vi "LabVIEW Final Project standard.vi"() -> ()   [LabVIEW 2022 SP3]
uses:
  <vilib>/sound2/lvsound2.llb/Sampling Mode.ctl
  <vilib>/Analysis/2dsp.llb/Real FFT.vi
  <vilib>/sound2/lvsound2.llb/Sound Input Read (DBL).vi
  <vilib>/measure/matone.llb/Extract Multiple Tone Information 1 Chan.vi
  <vilib>/Analysis/NI_AALPro.lvlib
  <vilib>/measure/NI_MAPro.lvlib
panel:
  out "multiple tone information":T1(array[cluster]) {"detected phase (deg)" format="%_6g"; "detected amplitude" format="%_6p"; "detected frequency" format="%_6p"}
  out "Spectrum":dbl[](graph)
  out "Original":dbl[](graph)
  in  "stop":bool
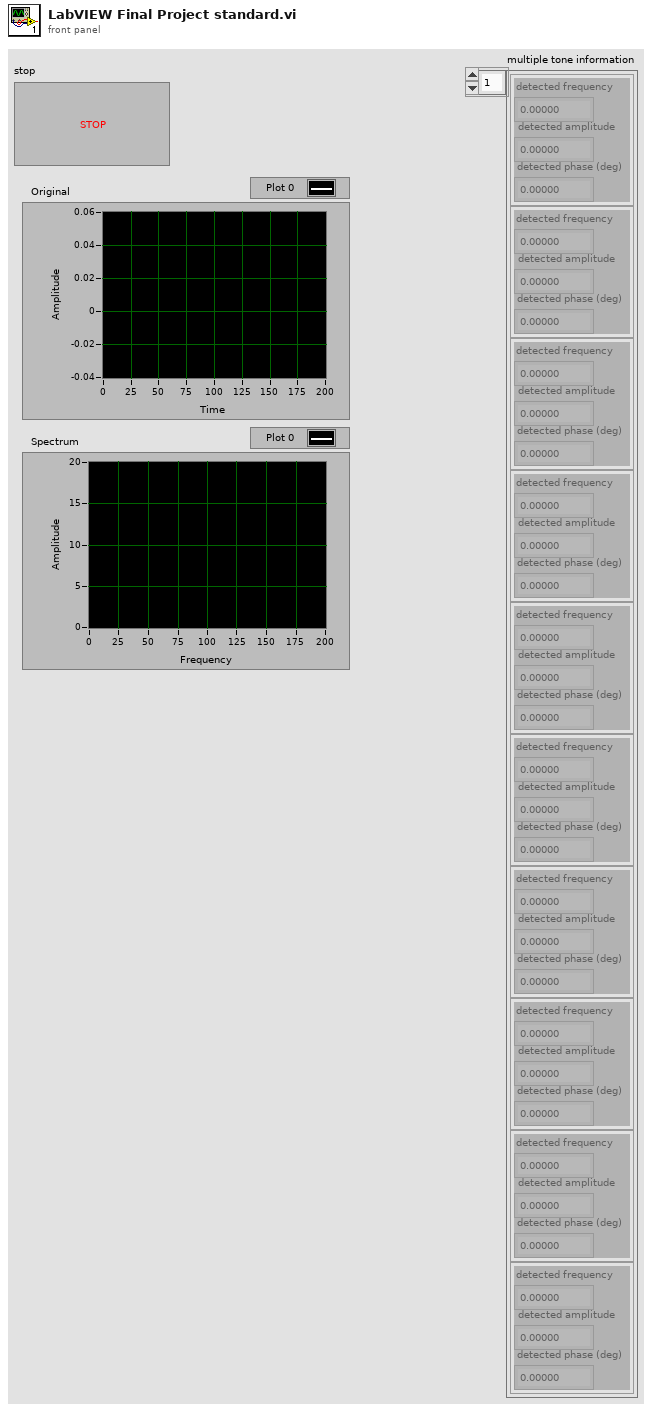
[diagram p1: front panel]
types:
  T1 = cluster{"detected frequency":dbl, "detected amplitude":dbl, "detected phase (deg)":dbl}[]
  T2 = enum32{"none", "input signal", "detected signal", "residual signal"}
  T3 = typedef "Sampling Mode.ctl" = i32
  T4 = typedef "Sound Input Task ID.ctl" = u32
  T5 = cluster{"detected frequency":dbl, "detected amplitude":dbl, "detected phase (deg)":dbl}
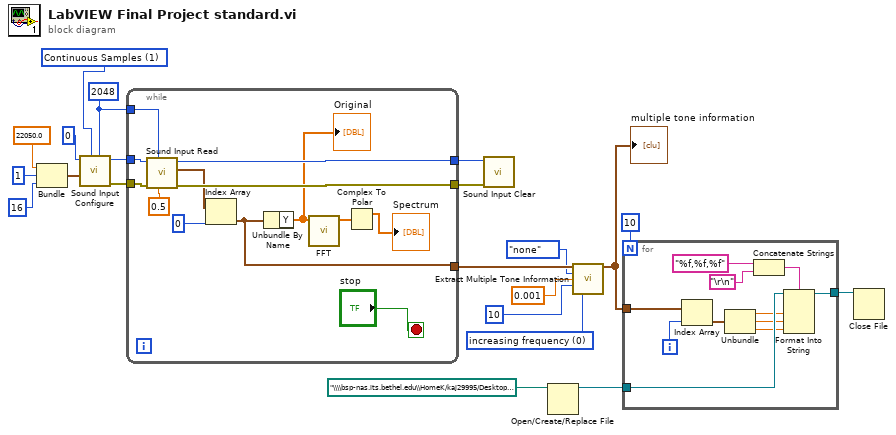
[diagram p0: block diagram]
diagram:
  w1 = 0 items=["increasing frequency", "decreasing amplitude"] ("output sorting")
  w13 = 2048 ("number of samples/ch")
  w16 = T3 1 items=["Finite Samples", "Continuous Samples"] ("sample mode")
  n1 = Bundle(22050.0, 1, 16) -> (w18:cluster{dbl, i32, i32})  [unwired: 1 in]
  n2 = call <vilib>:"Sound Input Configure.vi"("number of samples/ch"=w13, "sample mode"=w16, "sound format"=w18, "device ID"=u32 0) -> ("error out"=w15:errorcluster, "task ID"=w14:T4)  [unwired: 6 in]
  n3 = while {
    tunnel: w15 -> [w31]
    tunnel: w14 -> [w30]
    tunnel: w13 -> [w29]
    tunnel: [w28] -> w12
    tunnel: [w27] -> w11
    tunnel: [w22] -> w5
    stop <- "stop" stop-if-true
    n4 = call-poly <vilib>:"Sound Input Read.vi"("timeout (sec)"=0.5, "number of samples/ch"=w29, "error in (no error)"=w31, "task ID"=w30) -> ("error out"=w27:errorcluster, "data"=w24:waveform(dbl)[], "task ID out"=w28:T4)  [unwired: 5 in]
    n5 = Index Array(array=w24, index=0) -> (element=w22:waveform(dbl))
    n6 = Unbundle By Name(w22) -> ("Y"=w26:dbl[])
    "Original" <- w26
    n7 = call-poly <vilib>:"FFT.vi"("X"=w26) -> ("FFT {X}"=w25:cdb[])  [unwired: 9 in, 1 out]
    n8 = Complex To Polar(r * e^(i*theta)=w25) -> (r=→"Spectrum":dbl[])  [unwired: 1 out]
  }
  n9 = call <vilib>:"Sound Input Clear.vi"("error in (no error)"=w11, "task ID"=w12) -> ()  [unwired: 9 in, 1 out]
  n10 = Open/Create/Replace File(file path (use dialog)=path "\\\\bsp-nas.its.bethel.edu\\HomeK/kaj29995/Desktop/standardvoice.txt") -> (refnum out=w9:refnum<file>)  [unwired: 5 in, 2 out]
  n11 = call-poly <vilib>:"Extract Multiple Tone Information.vi"("time signal in"=w5, "export mode"=T2."none", "threshold"=0.001, "max num tones"=10, "output sorting"=w1) -> ("multiple tone information"=w6:T1)  [unwired: 8 in, 2 out]
  "multiple tone information" <- w6
  n12 = for {
    N: 10 -> [_]
    tunnel: w6 -> [w45]
    tunnel: w9 -> [w42]
    tunnel: [w41] -> w8
    i -> [w43]
    n13 = Index Array(array=w45, index=w43) -> (element=w44:T5)
    n14 = Unbundle(w44) -> ("detected frequency"=w40:dbl, "detected amplitude"=w39:dbl, "detected phase (deg)"=w38:dbl)
    n15 = Concatenate Strings("%f,%f,%f", "\r\n") -> (w36:string)
    n16 = Format Into String(format string=w36, initial string=w42, w40, w39, w38) -> (resulting string=w41:refnum<file>)  [unwired: 1 in, 1 out]
  }
  n17 = Close File(refnum=w8) -> ()  [unwired: 1 in, 2 out]
